vi "Configure Transform-CV.vi"(7 "cpu/gpu":enum32{"Item 0", "Item 1"}(ring), 8 "error in (no error)":errorcluster, 9 "model params":T1, 10 "classes":path, 11 "model":path) -> (0 "error out":errorcluster, 2 "model loaded?":bool, 3 "transformCvToolkit out":refnum<class "transformCv.lvclass">)   [LabVIEW 2024, in "transformCv.lvclass"]
uses:
  transformCv.lvclass
  modelParameters.ctl
  transformCv.lvclass/transformCv.ctl
  dependencies_dll_release/TCV_Lib.dll
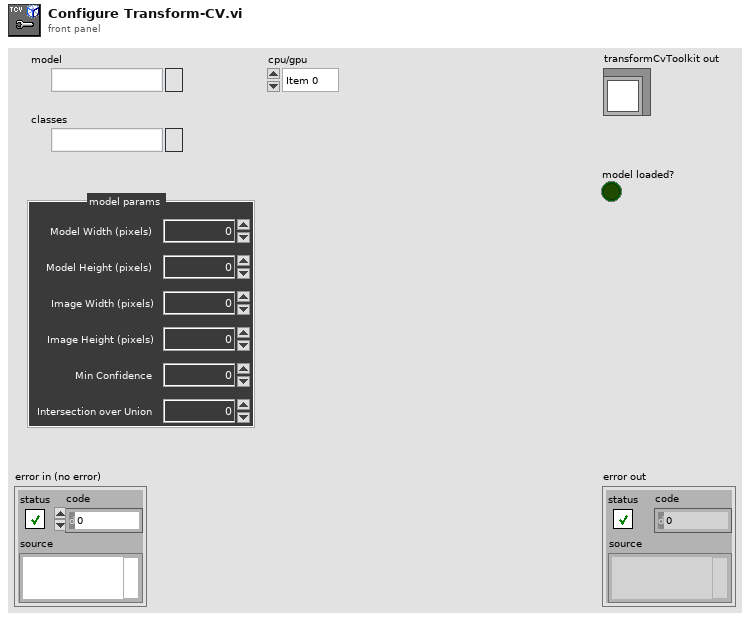
[diagram p1: front panel]
types:
  T1 = typedef "transformCv.lvclass/modelParameters.ctl" = cluster{"conf":dbl, "iou":dbl, "model w":i32, "model h":i32, "img w ":i32, "img h":i32}
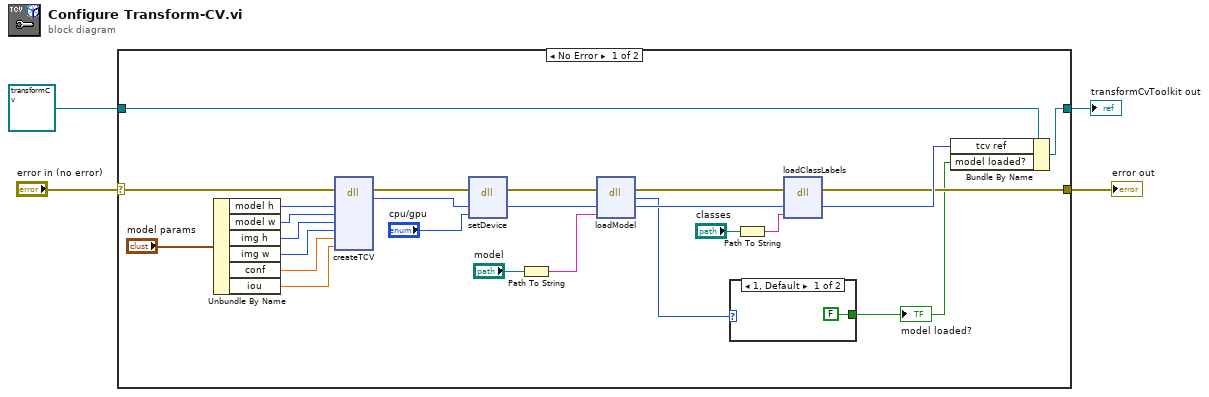
[diagram p0: block diagram]
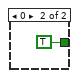
[diagram p2: hidden frame]
diagram:
  n1 = case shown="No Error" "error in (no error)" {
    selector: "error in (no error)" -> [w29 w33]
    tunnel: [w7 w33] -> w3
    tunnel: [w8 w32] -> w1
    tunnel: refnum<class "transformCv.lvclass"> refnum ("transformCvToolkit in") -> [w10 w32]
    frame No Error {
      n2 = Unbundle By Name("model params") -> ("model h"=w27:i32, "model w"=w26:i32, "img h"=w25:i32, "img w"=w24:i32, "conf"=w23:dbl, "iou"=w22:dbl)
      n3 = dll-call lib="C:/Users/jason/Documents/ads/tcv/TransformCV-LabVIEW/Test/dependencies_dll_release/TCV_Lib.dll" fn="createTCV"(error in=w29, "model_h"=w27, "model_w"=w26, "frame_h"=w25, "frame_w"=w24, "conf"=w23, "iou"=w22) -> (error out=w21:errorcluster, "return Obj"=w20:u64)  [unwired: 8 in, 1 out]
      n4 = dll-call lib="C:/Users/jason/Documents/ads/tcv/TransformCV-LabVIEW/Test/dependencies_dll_release/TCV_Lib.dll" fn="setDevice"(error in=w21, "ref"=w20, "device"="cpu/gpu") -> (error out=w18:errorcluster, "ref"=w11:u64)  [unwired: 4 in, 1 out]
      n5 = Path To String(path="model") -> (string=w15:string)
      n6 = dll-call lib="C:/Users/jason/Documents/ads/tcv/TransformCV-LabVIEW/Test/dependencies_dll_release/TCV_Lib.dll" fn="loadModel"(error in=w18, "ref"=w11, "path"=w15) -> (error out=w17:errorcluster, "success"=w6:i32, "ref"=w12:u64)  [unwired: 3 in, 1 out]
      n7 = case shown="1, Default" w6 {
        tunnel: [FALSE TRUE] -> w5
        frame 1, Default {
        }
        frame 0 {
        }
      }
      "model loaded?" <- w5
      n8 = Path To String(path="classes") -> (string=w13:string)
      n9 = dll-call lib="C:/Users/jason/Documents/ads/tcv/TransformCV-LabVIEW/Test/dependencies_dll_release/TCV_Lib.dll" fn="loadClassLabels"(error in=w17, "ref"=w12, "class_names"=w13) -> (error out=w7:errorcluster, "ref"=w9:u64)  [unwired: 4 in, 1 out]
      n10 = Bundle By Name(cluster=w10, "tcv ref"=w9, "model loaded?"=w5) -> (w8:refnum<class "transformCv.lvclass">)
    }
    frame Error {
    }
  }
  "error out" <- w3
  "transformCvToolkit out" <- w1
